vi "Fast Get Item Reference by Path FuncGlobal.vi"(5 "Action":enum16{"Open or Add", "Close Ref"}(ring), 8 "error in (no error)":errorcluster, 10 "Root Ref":T1=18446744073709551615 format="%.0x", 11 "Item Path in":string) -> (0 "error out":errorcluster, 2 "Item Ref":T1 format="%.0x", 3 "Item Path out":string, 4 "Found":bool)   [LabVIEW 2011]
doc: "Returns a reference to the item specified by <B>Item Path in</B>."
uses:
  <vilib>/NI Veristand/Custom Device API/Custom Device Item Ref.ctl
  <vilib>/NI Veristand/Custom Device API/Custom Device API.lvlib
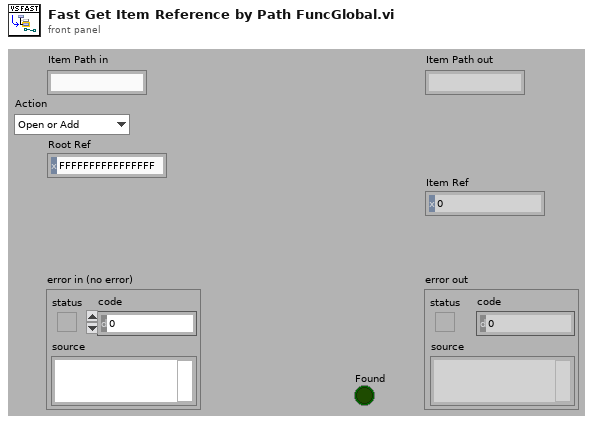
[diagram p1: front panel]
types:
  T1 = typedef "Custom Device API.lvlib/Custom Device Item Ref.ctl" = u64
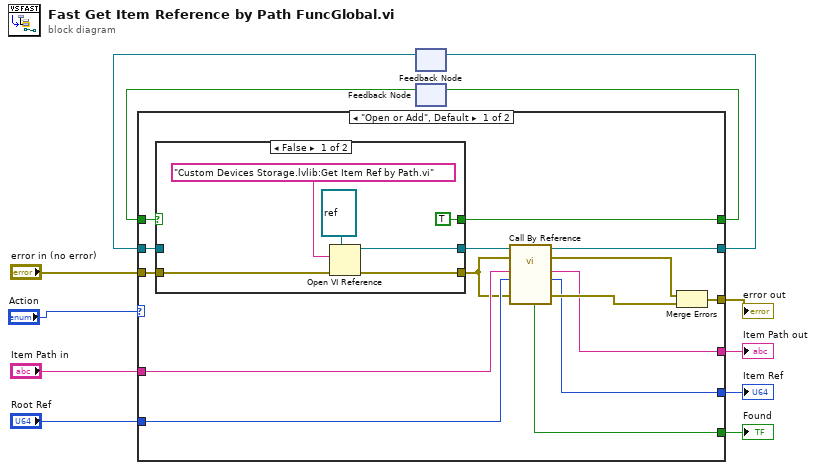
[diagram p0: block diagram]
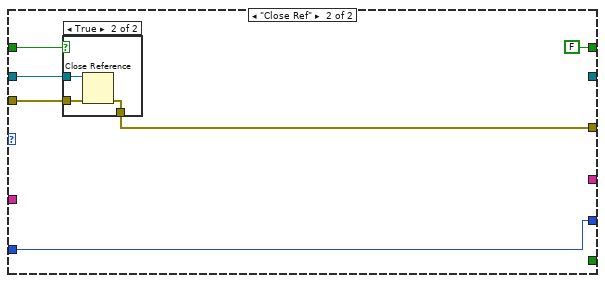
[diagram p3: hidden frame]
diagram:
  n1 = feedback #1() -> (w3:refnum<vi>)  [unwired: 1 in]
  n2 = feedback #2() -> (w4:bool)  [unwired: 1 in]
  n3 = case shown="\"Open or Add\", Default" "Action" {
    tunnel: [w26 _] -> w2
    tunnel: [w25 w39] -> w12
    tunnel: "Item Path in" -> [w24 _]
    tunnel: [w23 _] -> w10
    tunnel: [w22 w37] -> w9
    tunnel: [w21 _] -> w8
    tunnel: "error in (no error)" -> [w20 w40]
    tunnel: "Root Ref" -> [w19 w37]
    tunnel: [w15 FALSE] -> w5
    tunnel: w4 -> [w14 w42]
    tunnel: w3 -> [w13 w41]
    frame "Open or Add", Default {
      n4 = case shown="False" w14 {
        selector: w14 -> [_ w36]
        tunnel: w20 -> [w31 w34]
        tunnel: [w30 w35] -> w18
        tunnel: [w29 w34] -> w17
        tunnel: [TRUE w36] -> w15
        tunnel: w13 -> [_ w35]
        frame False {
          n5 = Open VI Reference(type specifier VI Refnum (for type only)=refnum<vi> refnum, vi path="Custom Devices Storage.lvlib:Get Item Ref by Path.vi", error in (no error)=w31) -> (vi reference=w30:refnum<vi>, error out=w29:errorcluster)  [unwired: 3 out]
        }
        frame True {
        }
      }
      n6 = call-by-ref "?"(reference=w18, error in=w17, 8:"error in (no error)"=w17, "Root Ref"=w19, "Item Path in"=w24) -> (reference out=w26:refnum<vi>, error out=w16:errorcluster, 0:"error out"=w27:errorcluster, "Item Ref"=w22:T1, "Item Path out"=w23:string, "Found"=w21:bool)  [unwired: 5 in]
      n7 = Merge Errors(w16, w27) -> (w25:errorcluster)
    }
    frame "Close Ref" {
      n8 = case shown="True" w42 {
        tunnel: w41 -> [_ w46]
        tunnel: w40 -> [w43 w45]
        tunnel: [w43 w44] -> w39
        frame False {
        }
        frame True {
          n9 = Close Reference(reference=w46, error in (no error)=w45) -> (error out=w44:errorcluster)
        }
      }
    }
  }
  "error out" <- w12
  "Found" <- w8
  "Item Ref" <- w9
  "Item Path out" <- w10
  n10 = feedback-in #1(w2) -> ()
  n11 = feedback-in #2(w5) -> ()
